vi "Register Events.vi"(8 "error in (no error)":errorcluster, 11 "Example Source in":refnum<class "Example Source.lvclass">) -> (0 "error out":errorcluster, 3 "Example Source out":refnum<class "Example Source.lvclass">)   [LabVIEW 2016, in "Example Source.lvlib" / "Example Source.lvclass"]
uses:
  Example Source.lvclass
  C:/Projects/Shared Libraries/Event Actors/Event Source/Event Source.lvclass
  Alternative Example Sink/Example Sink Messages/Update Array Msg/Update Array Msg.lvclass
  C:/Projects/Shared Libraries/Event Actors/Event Source Messages/Event Generated Msg/Event Generated Msg.lvclass
  Example Events/Double Array Event.lvclass
  C:/Projects/Shared Libraries/Event Actors/Event/Event.lvclass
  Alternative Example Sink/Example Sink Messages/Update Time Msg/Update Time Msg.lvclass
  Example Events/Timestamp Event.lvclass
  Alternative Example Sink/Example Sink Messages/Update Boolean Msg/Update Boolean Msg.lvclass
  Example Events/Boolean Event.lvclass
  Event/Event.lvclass/Event.ctl
  Example Sink/Example Sink Messages/Update Array Msg/Update Array Msg.lvclass
  Event/Event.lvclass
  Example Sink/Example Sink Messages/Update Time Msg/Update Time Msg.lvclass
  Event Source Messages/Register by Name Msg/Register by Name Msg.lvclass
  <vilib>/ActorFramework/Actor/Actor.lvclass
  Event Source/Event Source.lvclass
  C:/Program Files (x86)/National Instruments/LabVIEW 2016/vi.lib/ActorFramework/Actor/Actor.lvclass
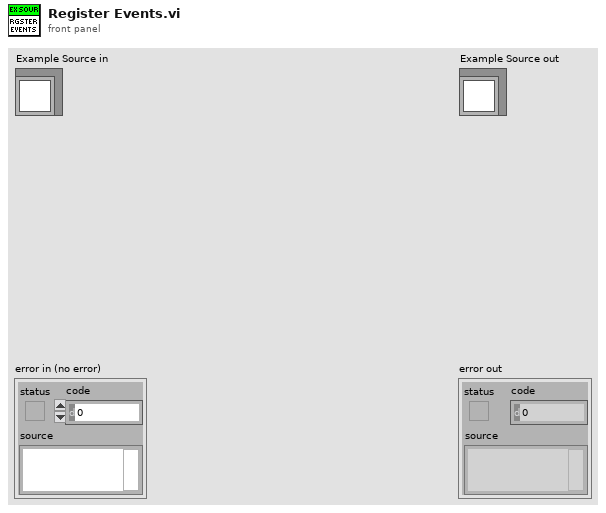
[diagram p1: front panel]
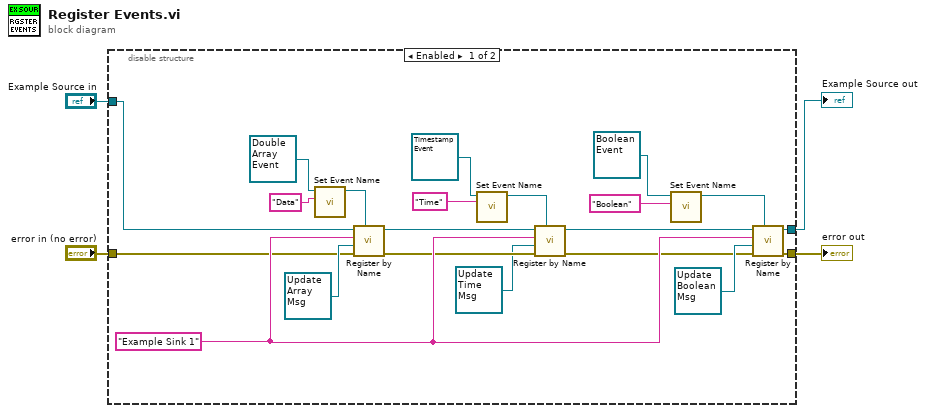
[diagram p0: block diagram]
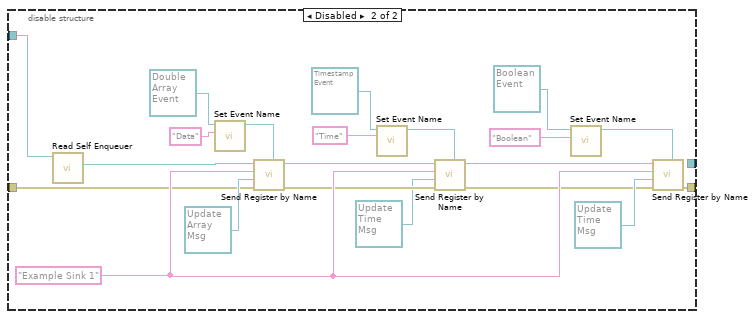
[diagram p2: hidden frame]
diagram:
  n1 = disable-structure shown="Enabled" {
    disable-tunnel: "Example Source in" -> [w10 w30]
    disable-tunnel: "error in (no error)" -> [w9 w29]
    disable-tunnel: [w8 w28] -> w2
    disable-tunnel: [w5 _] -> w1
    frame Enabled {
      w15 = "Example Sink 1" ("Debug Alias")
      n2 = call "Set Event Name.vi"("Name (Generic)"="Data", "Event In"=refnum<class "Double Array Event.lvclass"> refnum ("Double Array Event.lvclass")) -> ("Event Out"=w19:refnum<class "Double Array Event.lvclass">)  [unwired: 9 in]
      n3 = call "Register by Name.vi"("Event"=w19, "error in (no error)"=w9, "Event Fire Handler"=refnum<class "Update Array Msg.lvclass"> refnum ("Update Array Msg.lvclass"), "Sink Name"=w15, "Event Source in"=w10) -> ("error out"=w12:errorcluster, "Event Source out"=w14:refnum<class "Example Source.lvclass">)  [unwired: 5 in]
      n4 = call "Set Event Name.vi"("Name (Generic)"="Time", "Event In"=refnum<class "Timestamp Event.lvclass"> refnum ("Timestamp Event.lvclass")) -> ("Event Out"=w6:refnum<class "Timestamp Event.lvclass">)  [unwired: 9 in]
      n5 = call "Register by Name.vi"("Event"=w6, "error in (no error)"=w12, "Event Fire Handler"=refnum<class "Update Time Msg.lvclass"> refnum ("Update Time Msg.lvclass"), "Sink Name"=w15, "Event Source in"=w14) -> ("error out"=w11:errorcluster, "Event Source out"=w13:refnum<class "Example Source.lvclass">)  [unwired: 5 in]
      n6 = call "Set Event Name.vi"("Name (Generic)"="Boolean", "Event In"=refnum<class "Boolean Event.lvclass"> refnum ("Example Source.lvlib:Boolean Event.lvclass")) -> ("Event Out"=w17:refnum<class "Boolean Event.lvclass">)  [unwired: 9 in]
      n7 = call "Register by Name.vi"("Event"=w17, "error in (no error)"=w11, "Event Fire Handler"=refnum<class "Update Boolean Msg.lvclass"> refnum ("Update Time Msg.lvclass"), "Sink Name"=w15, "Event Source in"=w13) -> ("error out"=w8:errorcluster, "Event Source out"=w5:refnum<class "Example Source.lvclass">)  [unwired: 5 in]
    }
    frame Disabled {
      w36 = "Example Sink 1" ("Debug Alias")
      n8 = call <vilib>:"Read Self Enqueuer.vi"("Actor"=w30) -> ("Self Enqueuer"=w35:refnum<class "Message Enqueuer.lvclass">)  [unwired: 10 in]
      n9 = call "Set Event Name.vi"("Name (Generic)"="Data", "Event In"=refnum<class "Double Array Event.lvclass"> refnum ("Double Array Event.lvclass")) -> ("Event Out"=w40:refnum<class "Double Array Event.lvclass">)  [unwired: 9 in]
      n10 = call "Send Register by Name.vi"("Event"=w40, "error in (no error)"=w29, "Event Fire Handler"=refnum<class "Update Array Msg.lvclass"> refnum ("Update Array Msg.lvclass"), "Sink Name"=w36, "Message Enqueuer in"=w35) -> ("error out"=w32:errorcluster, "Message Enqueuer out"=w34:refnum<class "Message Enqueuer.lvclass">)  [unwired: 5 in]
      n11 = call "Set Event Name.vi"("Name (Generic)"="Time", "Event In"=refnum<class "Timestamp Event.lvclass"> refnum ("Timestamp Event.lvclass")) -> ("Event Out"=w26:refnum<class "Timestamp Event.lvclass">)  [unwired: 9 in]
      n12 = call "Send Register by Name.vi"("Event"=w26, "error in (no error)"=w32, "Event Fire Handler"=refnum<class "Update Time Msg.lvclass"> refnum ("Update Time Msg.lvclass"), "Sink Name"=w36, "Message Enqueuer in"=w34) -> ("error out"=w31:errorcluster, "Message Enqueuer out"=w33:refnum<class "Message Enqueuer.lvclass">)  [unwired: 5 in]
      n13 = call "Set Event Name.vi"("Name (Generic)"="Boolean", "Event In"=refnum<class "Boolean Event.lvclass"> refnum ("Example Source.lvlib:Boolean Event.lvclass")) -> ("Event Out"=w38:refnum<class "Boolean Event.lvclass">)  [unwired: 9 in]
      n14 = call "Send Register by Name.vi"("Event"=w38, "error in (no error)"=w31, "Event Fire Handler"=refnum<class "Update Time Msg.lvclass"> refnum ("Update Time Msg.lvclass"), "Sink Name"=w36, "Message Enqueuer in"=w33) -> ("error out"=w28:errorcluster)  [unwired: 5 in, 1 out]
    }
  }
  "error out" <- w2
  "Example Source out" <- w1
